vi "API Paths.vi"() -> (1 "API Folder":path, 2 "API Zip File":path)   [LabVIEW 2021]
doc: "Returns the paths to the installed API folder and the zip file it should be backed up to."
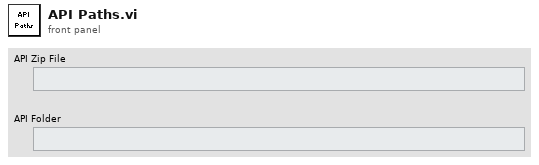
[diagram p1: front panel]
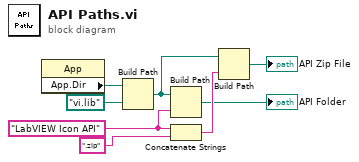
[diagram p0: block diagram]
diagram:
  w7 = "LabVIEW Icon API"
  n1 = property class="App"() -> ("App.Dir"=w1:path)  [unwired: 2 in, 2 out]
  n2 = Build Path(base path=w1, name or relative path=path "vi.lib" ("symbolic path")) -> (appended path=w5:path)
  n3 = Build Path(base path=w5, name or relative path=w7) -> (appended path=→"API Folder":path)
  n4 = Concatenate Strings(w7, ".zip" ("string")) -> (w4:string)
  n5 = Build Path(base path=w5, name or relative path=w4) -> (appended path=→"API Zip File":path)
